vi "Color_Project.vi"() -> ()   [LabVIEW 2013]
uses:
  leitura de dados txt control.ctl
  <vilib>/Utility/file.llb/Write To Spreadsheet File (DBL).vi
panel:
  out "L*a*b* 3":dbl[](array[numeric])
  out "XYZ":dbl[](array[numeric])
  out "RGB":dbl[](array[numeric])
  in  "C0":dbl min=0.0 max=1.0
  in  "RMix1":dbl[](array[numeric])
  in  "Selected RGB":string="0"
  in  "RMix2":dbl[](array[numeric])
  in  "Reflectance":dbl[](array[numeric])
  in  "Tab Control":T1(tab)
  in  "Create reflectance":bool
  in  "Nome da cor":string
  in  "SaveReflectance":bool
  out "Reflectance graph":cluster{"Value":dbl[], dbl[]}(graph) caption="Espectro de reflectância selecionado"
  in  "CalculateColor":bool
  in  "SelectReflectance":bool
  out "CMF graph":cluster{"X":dbl[], "Y":dbl[]}[](graph)
  in  "Select Illuminant":T2
  in  "Color Matching Function":string(combo)
  out "Iluminante Graph":cluster{"Value":dbl[], "Value":dbl[]}[](graph)
  out "Color":u32(colorbox)
  in  "780nm":dbl(slide)=0.05 min=0.01 max=0.99 scale=0.0..1.0 scale format="%1.3f"
  in  "700nm":dbl(slide)=0.05 min=0.01 max=0.99 scale=0.0..1.0 scale format="%1.3f"
  in  "650nm":dbl(slide)=0.05 min=0.01 max=0.99 scale=0.0..1.0 scale format="%1.3f"
  in  "575nm":dbl(slide)=0.05 min=0.01 max=0.99 scale=0.0..1.0 scale format="%1.3f"
  in  "550nm":dbl(slide)=0.05 min=0.01 max=0.99 scale=0.0..1.0 scale format="%1.3f"
  in  "525nm":dbl(slide)=0.05 min=0.01 max=0.99 scale=0.0..1.0 scale format="%1.3f"
  in  "500nm":dbl(slide)=0.05 min=0.01 max=0.99 scale=0.0..1.0 scale format="%1.3f"
  in  "600nm":dbl(slide)=0.05 min=0.01 max=0.99 scale=0.0..1.0 scale format="%1.3f"
  in  "450nm":dbl(slide)=0.05 min=0.01 max=0.99 scale=0.0..1.0 scale format="%1.3f"
  in  "380nm":dbl(slide)=0.05 min=0.01 max=0.99 scale=0.0..1.0 scale format="%1.3f"
  in  "Tab Control 3":enum32{"Misturar", "Estatísticas"}(tab)
  out "ColorRM":cluster{"Value":dbl[], "Mixtured colors":dbl[]}(graph) caption="Gráfico da reflectância das cores misturadas"
  in  "MixColors":bool
  in  "Selecione a concentração da cor 1":dbl(slide) scale=0.0..1.0 scale format="%#.4g"
  out "2000":dbl caption="Diferença: Cor 1 - Cor misturada"
  out "CD2-M":dbl caption="Diferença: Cor 2 - Cor misturada"
  out "L*a*b* MixedColor":dbl[](array[numeric]) caption="L*a*b* mixtura"
  out "L*a*b*":dbl[](array[numeric]) caption="L*a*b* cor 1"
  out "L*a*b* 2":dbl[](array[numeric]) caption="L*a*b* cor 2"
  out "Cor complementar":u32(colorbox)
  out "MixedColors":u32(colorbox) caption="Cor resultante"
  out "ColorR2":cluster{"Value":dbl[], "Mixtured colors":dbl[]}(graph) caption="Gráfico de reflectância da cor 2"
  out "ColorR1":cluster{"Value":dbl[], "Mixtured colors":dbl[]}(graph) caption="Gráfico de reflectância da cor 1"
  out "Color2":u32(colorbox) caption="Cor selecionada"
  out "Color1":u32(colorbox) caption="Cor selecionada"
  in  "SelectColor2":bool
  in  "SelectColor1":bool
  in  "Color Matching Function 2":string(combo) caption="Selecione o CMF"
  in  "SelectIlluminant2":T2 caption="Selecione o iluminante"
  out "Color1Complementar":u32(colorbox) caption="Cor complementar"
  out "Cor complementar  2":u32(colorbox) caption="Cor complementar"
  in  "SelectColor2":bool
  in  "SelectColor1":bool
  in  "Tab Control 2":enum32{"L*", "a*", "b*"}(tab)
  out "Componente L*":cluster{"X":dbl[], "L*a*b intermediary":dbl[]}(graph)
  out "Componente a*":cluster{"X":dbl[], "L*a*b intermediary":dbl[]}(graph)
  out "Componente b*":cluster{"X":dbl[], "L*a*b intermediary":dbl[]}(graph)
  in  "Color Matching Function 3":string(combo) caption="Selecione o CMF"
  in  "SelectIlluminant2 2":T2 caption="Selecione o iluminante"
  in  "Colors":u32[](array[colorbox])
  out "Espectros de reflectância referentes as cores intermediárias obtidas":cluster{"X":dbl[], "Y":dbl[]}[](graph)
  in  "MixByConcentration":bool
  in  "Mixed":dbl[](array[numeric])
  in  "MixByColorDifference":bool
  out "Color1 2":u32
  out "Color2 2":u32
  in  "C1":dbl=0.1 min=0.0 max=1.0
  in  "DeltaLabel":string[](array[string]) caption="Delta E"
  in  "ConcentrationLabel":string[](array[string]) caption="Concentração"
  out "teste":i32[](array[numeric])
  out "IL Table":string[][](array[string])
  out "ILCols":i32
  out "ILRows":i32
  out "Selected illuminant value":dbl[](array[numeric])
  out "Is CMF selected?":bool
  out "Is illuminant selected?":bool
  out "CMF Table":string[][](array[string])
  out "NeedInterpolation?":bool
  out "WhiteReference":i32[](array[numeric])
  out "Intepoled iluminants":dbl[][](array[numeric])
  out "Selected\nCMF":dbl[][](array[numeric])
  out "cmf Index":dbl
  out "CMFCols":i32
  out "CMFRows":i32
  out "LambdaInterval":dbl[](array[numeric])
  out "Selected illuminant index":dbl
  out "Selected illuminant NV":cluster{"Value":string, dbl[]}
  # "Primeira etapa - Seleção da iluminação desejada"
  # "Segunda etapa - Seleção do estímulo ocular do observador"
  # "Terceira etapa - Seleção ou criação de espectros de reflectância"
  # "Selecione o CMF"
  # "Selecione o iluminante"
  # "Etapa final - Calcular cor referente aos espectros"
  # "Sistema para criação de espectros de reflectância"
  # "Etapa básica - Seleção de iluminação e estímulos oculares"
  # "Etapa final - Calcular a mistura das cores e dosar a concentração da cor referência"
  # "Segunda etapa - Selecionar as cores desejadas para efetuar a mistura"
  # "Desvios de cor"
  # "Coordenadas de cor"
  # "Nesta seção serão avaliadas diferentes maneiras para misturas de cores:\n1 - Por variação de concentração\n2 - Por variação de desvio de cor"
  # "Análise de variação das componentes L*a*b* das cores geradas"
  # "Seleção de componentes"
  # "Seleção do tipo da mistura a ser efetuado"
  # "Representação das cores intermediárias gerada a partir\ndas misturas,e seus respectivos desvios e concentrações"
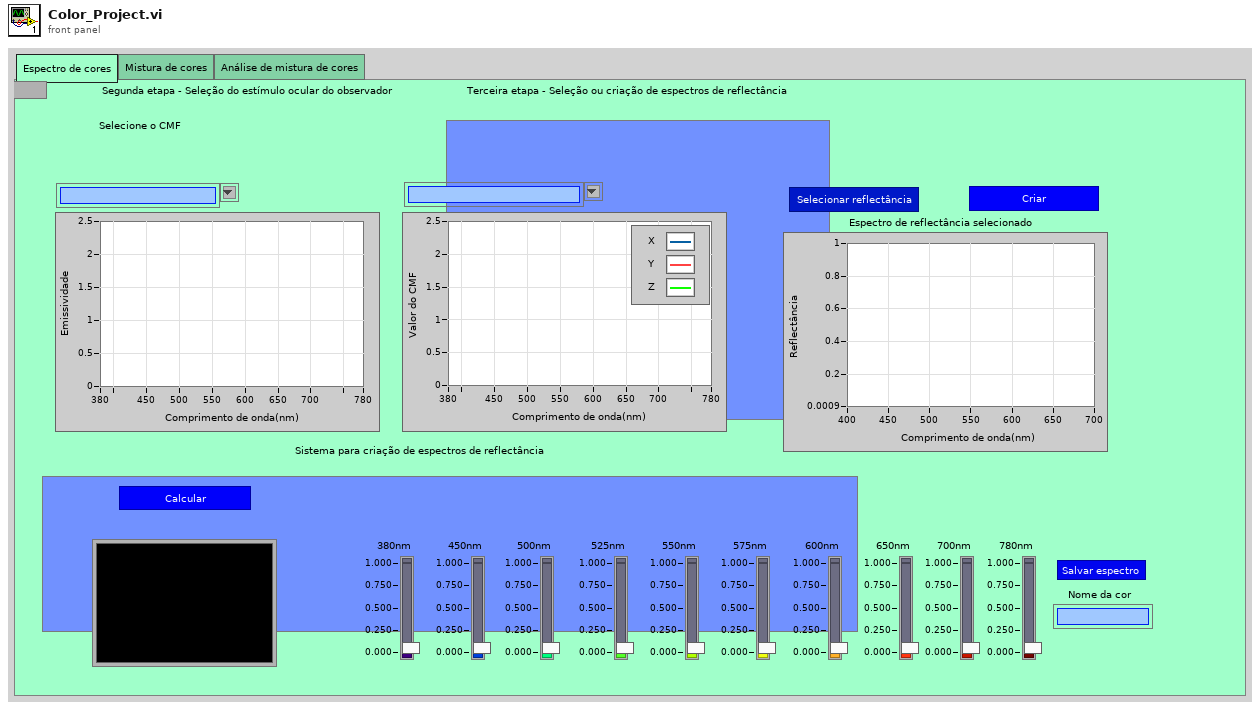
[diagram p1: front panel]
types:
  T1 = enum32{"Espectro de cores", "Mistura de cores", "Análise de mistura de cores"}
  T2 = typedef "leitura de dados txt control.ctl" = string
  T3 = cluster{"Value":cluster{"Value":string, dbl[]}, "Selected RGB":string, "Value":dbl[][]}
  T4 = cluster{"Color":u32, "RGB":dbl[], "L*a*b*":dbl[], "XYZ":dbl[]}
  T5 = cluster{cluster{i32[], dbl[]}, cluster{i32[], dbl[]}, cluster{i32[], dbl[]}}
  T6 = cluster{cluster{"X":dbl[], "L*a*b intermediary":dbl[]}, cluster{"X":dbl[], "L*a*b intermediary":dbl[]}, cluster{"X":dbl[], "L*a*b intermediary":dbl[]}}
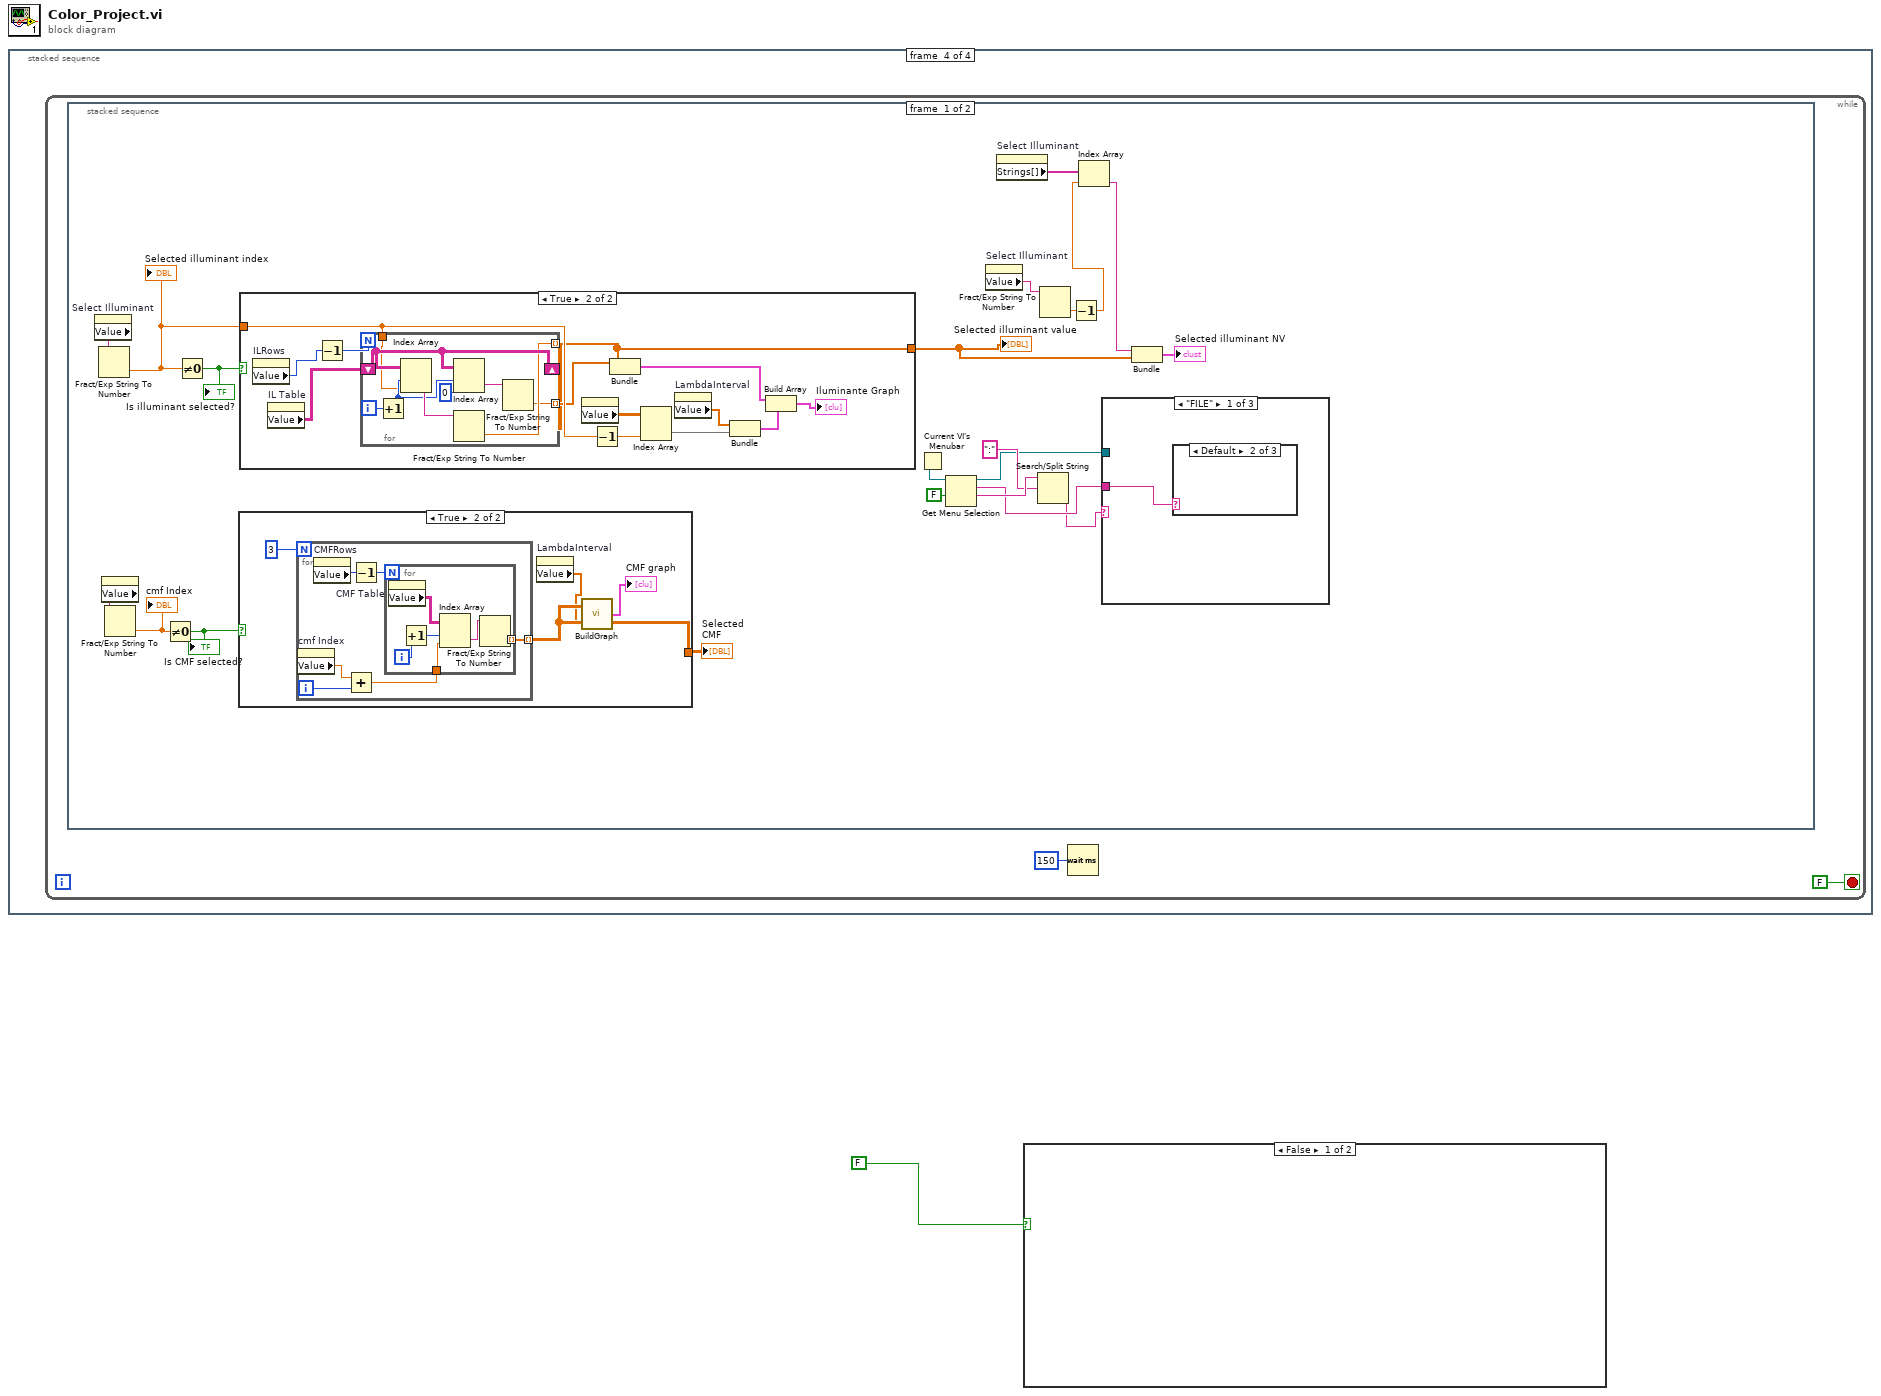
[diagram p0: block diagram]
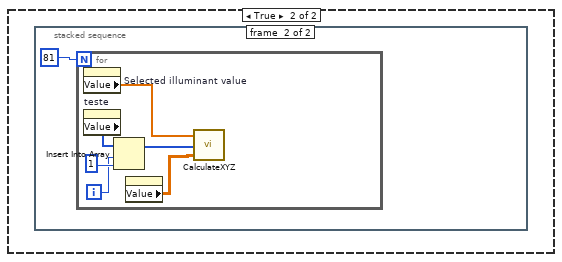
[diagram p2: hidden frame]
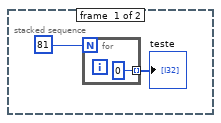
[diagram p3: hidden frame]
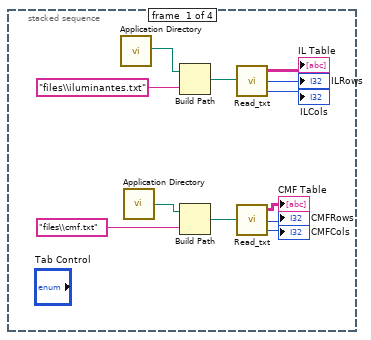
[diagram p4: hidden frame]
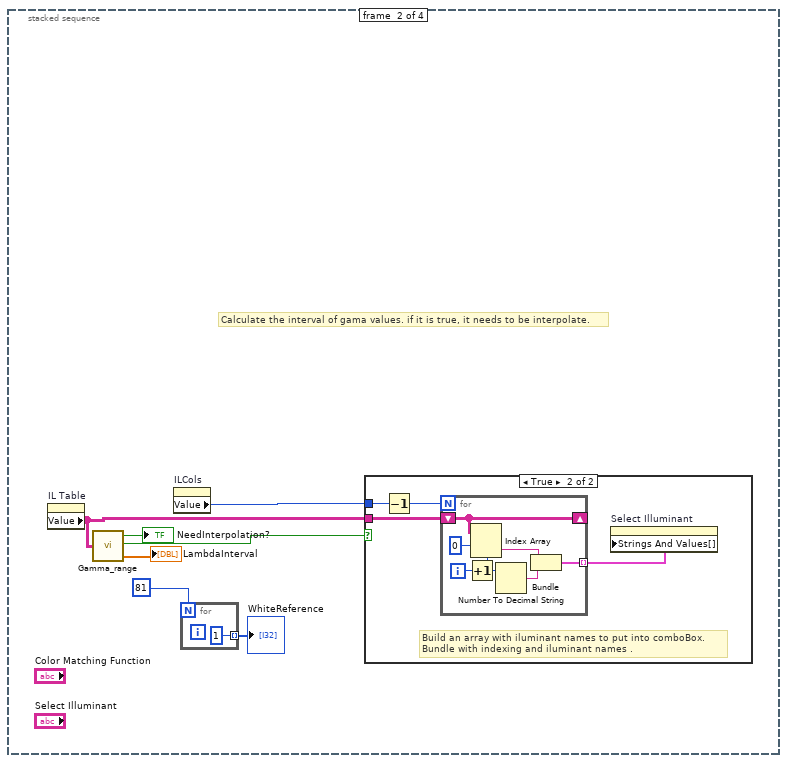
[diagram p5: hidden frame]
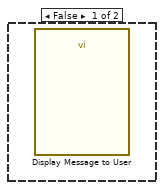
[diagram p6: hidden frame]
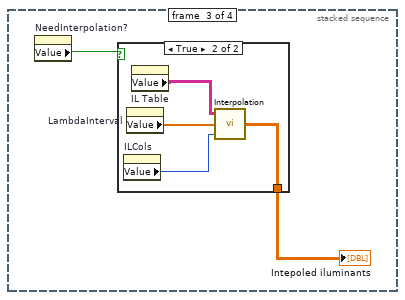
[diagram p7: hidden frame]
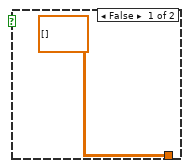
[diagram p8: hidden frame]
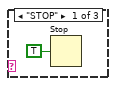
[diagram p9: hidden frame]
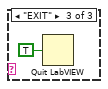
[diagram p10: hidden frame]
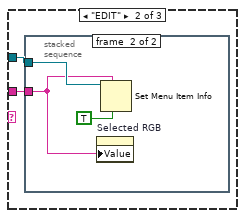
[diagram p11: hidden frame]
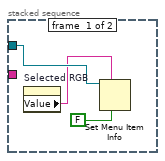
[diagram p12: hidden frame]
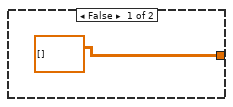
[diagram p14: hidden frame]
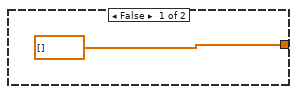
[diagram p15: hidden frame]
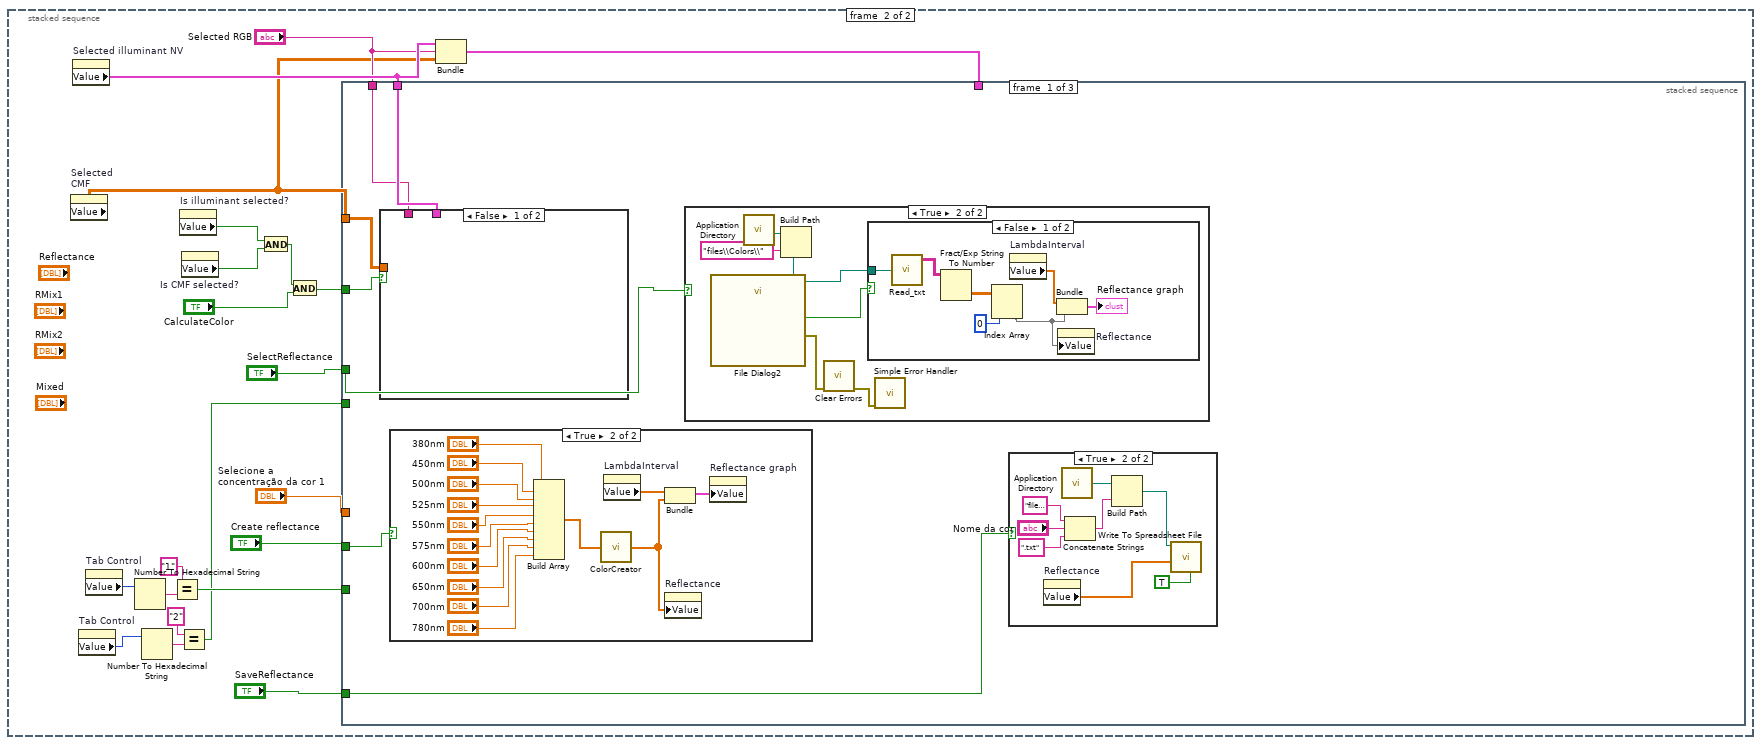
[diagram p16: hidden frame]
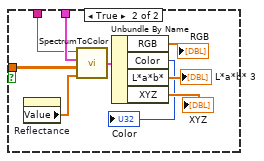
[diagram p18: hidden frame]
diagram:
  n1 = stacked-sequence {
    frame #0 {
      n2 = call <vilib>:"Application Directory.vi"() -> ("Application Directory"=w3:path)
      n3 = call <vilib>:"Application Directory.vi"() -> ("Application Directory"=w2:path)
      n4 = Build Path(base path=w3, name or relative path="files\\iluminantes.txt") -> (appended path=w5:path)
      n5 = Build Path(base path=w2, name or relative path="files\\cmf.txt") -> (appended path=w4:path)
      n6 = call "Read_txt.vi"("file path (dialog if empty)"=w5) -> ("Elements"=→"IL Table":string[][], "Rows"=→"ILRows":i32, "Cols"=→"ILCols":i32)
      n7 = call "Read_txt.vi"("file path (dialog if empty)"=w4) -> ("Elements"=→"CMF Table":string[][], "Rows"=→"CMFRows":i32, "Cols"=→"CMFCols":i32)
    }
    frame #1 {
      # "Calculate the interval of gama values. if it is true, it needs to be interpolate."
      n8 = property on="IL Table" class="Arr (strict)"() -> ("Value"=w15:string[][])  [unwired: 2 in, 2 out]
      n9 = call "Gamma_range.vi"("Illuminant Table"=w15) -> ("Interpolate"=→"NeedInterpolation?":bool, "In range?"=w17:bool, "GammaInterval"=→"LambdaInterval":dbl[])
      n10 = property on="ILCols" class="DigNum (strict)"() -> ("Value"=w18:i32)  [unwired: 2 in, 2 out]
      n11 = for {
        N: 81 -> [_]
        tunnel: [1] -> w19 mode=indexing
      }
      "WhiteReference" <- w19
      n12 = case shown="True" w17 {
        tunnel: w15 -> [_ w21]
        tunnel: w18 -> [_ w22]
        frame False {
          n13 = call "Display Message to User"() -> ()  [unwired: 10 in, 2 out]
        }
        frame True {
          # "Build an array with iluminant names to put into comboBox.\nBundle with indexing and iluminant names ."
          n14 = Decrement(x=w22) -> (x-1=w24:i32)
          n15 = for {
            N: w24 -> [_]
            shift-right: [w29] -> _
            shift-left: w21 -> [w29]
            tunnel: [w25] -> w23 mode=indexing
            i -> [w31]
            n16 = Increment(x=w31) -> (x+1=w28:i32)
            n17 = Index Array(array=w29, index (row)=0, index (col)=w28) -> (element=w26:string)
            n18 = Number To Decimal String(number=w28) -> (decimal integer string=w27:string)  [unwired: 1 in]
            n19 = Bundle("String"=w26, w27) -> (w25:cluster{"String":string, string})  [unwired: 1 in]
          }
          n20 = property on="Select Illuminant" class="CmbBox (strict)"("Strings And Values[]"=w23) -> ()  [unwired: 2 in, 2 out]
        }
      }
    }
    frame #2 {
      n21 = property on="NeedInterpolation?" class="Bool (strict)"() -> ("Value"=w34:bool)  [unwired: 2 in, 2 out]
      n22 = case shown="True" w34 {
        tunnel: [dbl[][] [] w38] -> w33
        frame False {
        }
        frame True {
          n23 = property on="ILCols" class="DigNum (strict)"() -> ("Value"=w36:i32)  [unwired: 2 in, 2 out]
          n24 = property on="LambdaInterval" class="Arr (strict)"() -> ("Value"=w39:dbl[])  [unwired: 2 in, 2 out]
          n25 = property on="IL Table" class="Arr (strict)"() -> ("Value"=w37:string[][])  [unwired: 2 in, 2 out]
          n26 = call "Interpolation.vi"("Number of Columns"=w36, "Lambda Interval"=w39, "Illuminants"=w37) -> ("Interpolated"=w38:dbl[][])
        }
      }
      "Intepoled iluminants" <- w33
    }
    frame #3 {
      n27 = while {
        stop <- FALSE stop-if-true
        n28 = stacked-sequence {
          frame #0 {
            n29 = property on="Select Illuminant" class="CmbBox (strict)"() -> ("Value"=w58:T2)  [unwired: 2 in, 2 out]
            n30 = Fract/Exp String To Number(string=w58) -> (number=w57:dbl)  [unwired: 3 in, 1 out]
            "Selected illuminant index" <- w57
            n31 = property on="Color Matching Function" class="CmbBox"() -> ("Value"=w60:string)  [unwired: 2 in, 2 out]
            n32 = Fract/Exp String To Number(string=w60) -> (number=w61:dbl)  [unwired: 3 in, 1 out]
            "cmf Index" <- w61
            n33 = Not Equal To 0?(x=w61) -> (x != 0?=w59:bool)
            "Is CMF selected?" <- w59
            n34 = Not Equal To 0?(x=w57) -> (x != 0?=w62:bool)
            "Is illuminant selected?" <- w62
            n35 = case shown="True" w59 {
              tunnel: [dbl[][] [] w77] -> w56
              frame False {
              }
              frame True {
                n36 = for {
                  N: 3 -> [_]
                  tunnel: [w81] -> w77 mode=indexing
                  i -> [w83]
                  n37 = property on="cmf Index" class="DigNum (strict)"() -> ("Value"=w84:dbl)  [unwired: 2 in, 2 out]
                  n38 = property on="CMFRows" class="DigNum (strict)"() -> ("Value"=w80:i32)  [unwired: 2 in, 2 out]
                  n39 = Add(x=w84, y=w83) -> (x+y=w82:dbl)
                  n40 = Decrement(x=w80) -> (x-1=w79:i32)
                  n41 = for {
                    N: w79 -> [_]
                    tunnel: w82 -> [w89]
                    tunnel: [w85] -> w81 mode=indexing
                    i -> [w88]
                    n42 = property on="CMF Table" class="Arr (strict)"() -> ("Value"=w90:string[][])  [unwired: 2 in, 2 out]
                    n43 = Increment(x=w88) -> (x+1=w87:i32)
                    n44 = Index Array(array=w90, index (row)=w87, index (col)=w89) -> (element=w86:string)
                    n45 = Fract/Exp String To Number(string=w86) -> (number=w85:dbl)  [unwired: 3 in, 1 out]
                  }
                }
                n46 = property on="LambdaInterval" class="Arr (strict)"() -> ("Value"=w76:dbl[])  [unwired: 2 in, 2 out]
                n47 = call "BuildGraph.vi"("X"=w76, "Y"=w77) -> ("Graph"=→"CMF graph":cluster{"X":dbl[], "Y":dbl[]}[])
              }
            }
            "Selected\nCMF" <- w56
            n48 = case shown="True" w62 {
              tunnel: w57 -> [_ w101]
              tunnel: [dbl[] [] w95] -> w55
              frame False {
              }
              frame True {
                n49 = property on="ILRows" class="DigNum (strict)"() -> ("Value"=w94:i32)  [unwired: 2 in, 2 out]
                n50 = property on="IL Table" class="Arr (strict)"() -> ("Value"=w93:string[][])  [unwired: 2 in, 2 out]
                n51 = Decrement(x=w94) -> (x-1=w104:i32)
                n52 = for {
                  N: w104 -> [_]
                  shift-right: [w112] -> _
                  shift-left: w93 -> [w112]
                  tunnel: w101 -> [w105]
                  tunnel: [w107] -> w95 mode=indexing
                  tunnel: [w106] -> w97 mode=indexing
                  i -> [w113]
                  n53 = Increment(x=w113) -> (x+1=w108:i32)
                  n54 = Index Array(array=w112, index (row)=w108, index (col)=w105) -> (element=w109:string)
                  n55 = Index Array(array=w112, index (row)=w108, index (col)=0 ("disabled index (col)")) -> (element=w110:string)
                  n56 = Fract/Exp String To Number(string=w109) -> (number=w107:dbl)  [unwired: 3 in, 1 out]
                  n57 = Fract/Exp String To Number(string=w110) -> (number=w106:dbl)  [unwired: 3 in, 1 out]
                }
                n58 = property on="Intepoled iluminants" class="Arr (strict)"() -> ("Value"=w99:dbl[][])  [unwired: 2 in, 2 out]
                n59 = Decrement(x=w101) -> (x-1=w100:dbl)
                n60 = Bundle(w97, w95) -> (w102:cluster{dbl[], dbl[]})  [unwired: 1 in]
                n61 = Index Array(array=w99, index (col)=w100) -> (element=w96:dbl[])  [unwired: 1 in]
                n62 = property on="LambdaInterval" class="Arr (strict)"() -> ("Value"=w98:dbl[])  [unwired: 2 in, 2 out]
                n63 = Bundle("Value"=w98, "Value"=w96) -> (w103:cluster{"Value":dbl[], "Value":dbl[]})  [unwired: 1 in]
                n64 = Build Array(w102, w103) -> (→"Iluminante Graph":cluster{"Value":dbl[], "Value":dbl[]}[])
              }
            }
            "Selected illuminant value" <- w55
            n65 = Current VI's Menubar() -> (w42:refnum<k9>)
            n66 = Get Menu Selection(0:w42, 2:FALSE ("block menu (F)")) -> (5:w45:refnum<k9>, 6:w44:string, 7:w47:string)  [unwired: 2 in, 2 out]
            n67 = property on="Select Illuminant" class="CmbBox (strict)"() -> ("Value"=w51:T2)  [unwired: 2 in, 2 out]
            n68 = property on="Select Illuminant" class="CmbBox (strict)"() -> ("Strings[]"=w53:string[])  [unwired: 2 in, 2 out]
            n69 = Search/Split String(string=w47, search string/char (-)=":") -> (substring before match=w43:string)  [unwired: 1 in, 2 out]
            n70 = Fract/Exp String To Number(string=w51) -> (number=w50:dbl)  [unwired: 3 in, 1 out]
            n71 = Decrement(x=w50) -> (x-1=w49:dbl)
            n72 = Index Array(array=w53, index=w49) -> (element=w52:string)
            n73 = case shown="\"FILE\"" w43 {
              tunnel: w45 -> [_ w67 _]
              tunnel: w44 -> [w63 w66 _]
              frame "FILE" {
                n74 = case shown="Default" w63 {
                  frame "STOP" {
                    n75 = Stop(stop? (T)=TRUE) -> ()
                  }
                  frame Default {
                  }
                  frame "EXIT" {
                    n76 = Quit LabVIEW(quit? (T)=TRUE) -> ()
                  }
                }
              }
              frame "EDIT" {
                n77 = stacked-sequence {
                  tunnel: w67 -> [w70 w73]
                  tunnel: w66 -> [_ w72]
                  frame #0 {
                    n78 = property on="Selected RGB" class="Str"() -> ("Value"=w68:string)  [unwired: 2 in, 2 out]
                    n79 = Set Menu Item Info(6:FALSE ("enabled"), 7:w68, 11:w70) -> ()  [unwired: 4 in, 2 out]
                  }
                  frame #1 {
                    n80 = property on="Selected RGB" class="Str"("Value"=w72) -> ()  [unwired: 2 in, 2 out]
                    n81 = Set Menu Item Info(6:TRUE ("enabled"), 7:w72, 11:w73) -> ()  [unwired: 4 in, 2 out]
                  }
                }
              }
              frame Default {
              }
            }
            n82 = Bundle(w52, w55) -> (→"Selected illuminant NV":cluster{string, dbl[]})  [unwired: 1 in]
          }
          frame #1 {
            n83 = property on="Selected\nCMF" class="Arr (strict)"() -> ("Value"=w125:dbl[][])  [unwired: 2 in, 2 out]
            n84 = property on="Selected illuminant NV" class="Clust (strict)"() -> ("Value"=w127:cluster{"Value":string, dbl[]})  [unwired: 2 in, 2 out]
            n85 = property on="Tab Control" class="TabCtl (strict)"() -> ("Value"=w118:T1)  [unwired: 2 in, 2 out]
            n86 = property on="Tab Control" class="TabCtl (strict)"() -> ("Value"=w121:T1)  [unwired: 2 in, 2 out]
            n87 = Number To Hexadecimal String(2:w121) -> (0:w122:string)  [unwired: 1 in]
            n88 = Number To Hexadecimal String(2:w118) -> (0:w119:string)  [unwired: 1 in]
            n89 = Equal?(x="1", y=w122) -> (x = y?=w120:bool)
            n90 = Equal?(x="2", y=w119) -> (x = y?=w116:bool)
            n91 = property on="Is illuminant selected?" class="Bool (strict)"() -> ("Value"=w132:bool)  [unwired: 2 in, 2 out]
            n92 = property on="Is CMF selected?" class="Bool (strict)"() -> ("Value"=w133:bool)  [unwired: 2 in, 2 out]
            n93 = And(x=w132, y=w133) -> (x .and. y?=w114:bool)
            n94 = And(x=w114, y="CalculateColor") -> (x .and. y?=w131:bool)
            n95 = Bundle("Value"=w127, "Selected RGB"="Selected RGB", "Value"=w125) -> (w124:T3)  [unwired: 1 in]
            n96 = stacked-sequence {
              tunnel: w127 -> [w139 w189 w248]
              tunnel: w125 -> [w138 w188 w247]
              tunnel: w131 -> [w137 _ _]
              tunnel: "SelectReflectance" -> [w141 _ _]
              tunnel: "Create reflectance" -> [w140 _ _]
              tunnel: "Selected RGB" -> [w136 w190 w249]
              tunnel: "Selecione a concentração da cor 1" -> [_ w191 _]
              tunnel: "SaveReflectance" -> [w135 _ _]
              tunnel: w124 -> [_ _ w246]
              tunnel: w120 -> [_ w187 _]
              tunnel: w116 -> [_ _ w245]
              frame #0 {
                n97 = case shown="False" w137 {
                  tunnel: w139 -> [_ w157]
                  tunnel: w138 -> [_ w156]
                  tunnel: w136 -> [_ w154]
                  frame False {
                  }
                  frame True {
                    n98 = property on="Reflectance" class="Arr (strict)"() -> ("Value"=w155:dbl[])  [unwired: 2 in, 2 out]
                    n99 = call "SpectrumToColor.vi"("Reflectance"=w155, "CMF"=w156, "Illuminant"=w157, "Selected RGB"=w154) -> ("Color,XYZ,RGB,Lab"=w158:T4)
                    n100 = Unbundle By Name(w158) -> ("RGB"=→"RGB":dbl[], "Color"=→"Color":u32, "L*a*b*"=→"L*a*b* 3":dbl[], "XYZ"=→"XYZ":dbl[])
                  }
                }
                n101 = case shown="True" w140 {
                  frame False {
                  }
                  frame True {
                    n102 = Build Array("380nm", "450nm", "500nm", "525nm", "550nm", "575nm", "600nm", "650nm", "700nm", "780nm") -> (w162:dbl[])
                    n103 = call "ColorCreator.vi"("Reflectance values"=w162) -> ("Spectrum"=w159:dbl[])
                    n104 = property on="LambdaInterval" class="Arr (strict)"() -> ("Value"=w160:dbl[])  [unwired: 2 in, 2 out]
                    n105 = Bundle("Value"=w160, "Spectrum"=w159) -> (w161:cluster{"Value":dbl[], "Spectrum":dbl[]})  [unwired: 1 in]
                    n106 = property on="Reflectance" class="Arr (strict)"("Value"=w159) -> ()  [unwired: 2 in, 2 out]
                    n107 = property on="Reflectance graph" class="XYGraph (strict)"("Value"=w161) -> ()  [unwired: 2 in, 2 out]
                  }
                }
                n108 = case shown="True" w141 {
                  frame False {
                  }
                  frame True {
                    n109 = call <vilib>:"Application Directory.vi"() -> ("Application Directory"=w178:path)
                    n110 = Build Path(base path=w178, name or relative path="files\\Colors\\") -> (appended path=w177:path)
                    n111 = call "File Dialog2"("start path"=w177) -> ("selected path"=w175:path, "cancelled"=w176:bool, "error out"=w174:errorcluster)  [unwired: 11 in, 1 out]
                    n112 = call <vilib>:"Clear Errors.vi"("error in (no error)"=w174) -> ("error out"=w173:errorcluster)  [unwired: 6 in]
                    n113 = case shown="False" w176 {
                      tunnel: w175 -> [w181 _]
                      frame False {
                        n114 = call "Read_txt.vi"("file path (dialog if empty)"=w181) -> ("Elements"=w186:string[][])  [unwired: 2 out]
                        n115 = Fract/Exp String To Number(string=w186) -> (number=w185:dbl[][])  [unwired: 3 in, 1 out]
                        n116 = Index Array(array=w185, index (col)=0 ("index (row)")) -> (element=w180:dbl[])  [unwired: 1 in]
                        n117 = property on="LambdaInterval" class="Arr (strict)"() -> ("Value"=w183:dbl[])  [unwired: 2 in, 2 out]
                        n118 = Bundle("Value"=w183, w180) -> (→"Reflectance graph":cluster{"Value":dbl[], dbl[]})  [unwired: 1 in]
                        n119 = property on="Reflectance" class="Arr (strict)"("Value"=w180) -> ()  [unwired: 2 in, 2 out]
                      }
                      frame True {
                        n120 = call "Display Message to User2"() -> ()  [unwired: 10 in, 2 out]
                      }
                    }
                    n121 = call <vilib>:"Simple Error Handler.vi"("error in (no error)"=w173) -> ()  [unwired: 4 in, 5 out]
                  }
                }
                n122 = case shown="True" w135 {
                  frame False {
                  }
                  frame True {
                    n123 = property on="Reflectance" class="Arr (strict)"() -> ("Value"=w147:dbl[])  [unwired: 2 in, 2 out]
                    n124 = call <vilib>:"Application Directory.vi"() -> ("Application Directory"=w149:path)
                    n125 = Concatenate Strings("files\\Colors\\" ("name or relative path"), "Nome da cor", ".txt") -> (w143:string)
                    n126 = Build Path(base path=w149, name or relative path=w143) -> (appended path=w148:path)
                    n127 = call-poly <vilib>:"Write To Spreadsheet File.vi"("transpose? (no:F)"=TRUE, "1D data"=w147, "file path (dialog if empty)"=w148) -> ()  [unwired: 5 in, 1 out]
                  }
                }
              }
              frame #1 {
                n128 = case shown="True" w187 {
                  tunnel: w191 -> [_ w206]
                  tunnel: w190 -> [_ w205]
                  tunnel: w189 -> [_ w204]
                  tunnel: w188 -> [_ w203]
                  frame False {
                  }
                  frame True {
                    n129 = property on="Color Matching Function" class="CmbBox"("Value"="Color Matching Function 2") -> ()  [unwired: 2 in, 2 out]
                    n130 = case shown="True" "MixColors" {
                      tunnel: w206 -> [_ w221]
                      frame False {
                      }
                      frame True {
                        n131 = property on="RMix2" class="Arr (strict)"() -> ("Value"=w222:dbl[])  [unwired: 2 in, 2 out]
                        n132 = property on="RMix1" class="Arr (strict)"() -> ("Value"=w211:dbl[])  [unwired: 2 in, 2 out]
                        n133 = call "ColorMixture.vi"("Concentration1"=w221, "Reflectance spectrum 2"=w222, "Reflectance spectrum"=w211) -> ("Mixtured colors"=w216:dbl[])  [unwired: 1 in]
                        n134 = property on="Selected illuminant NV" class="Clust (strict)"() -> (error out=w214:errorcluster, "Value"=w220:cluster{"Value":string, dbl[]})  [unwired: 2 in, 1 out]
                        n135 = property on="Selected\nCMF" class="Arr (strict)"() -> ("Value"=w219:dbl[][])  [unwired: 2 in, 2 out]
                        n136 = property on="LambdaInterval" class="Arr (strict)"() -> ("Value"=w217:dbl[])  [unwired: 2 in, 2 out]
                        n137 = property on="Selected RGB" class="Str"(error in=w214) -> ("Value"=w213:string)  [unwired: 1 in, 2 out]
                        n138 = call "SpectrumToColor.vi"("Reflectance"=w216, "CMF"=w219, "Illuminant"=w220, "Selected RGB"=w213) -> ("Color,XYZ,RGB,Lab"=w218:T4)
                        n139 = Bundle("Value"=w217, "Mixtured colors"=w216) -> (→"ColorRM":cluster{"Value":dbl[], "Mixtured colors":dbl[]})  [unwired: 1 in]
                        n140 = Unbundle By Name(w218) -> ("Color"=w208:u32, "L*a*b*"=→"L*a*b* MixedColor":dbl[], "RGB"=w210:dbl[])
                        "MixedColors" <- w208
                        n141 = call "RGBtoComplementar.vi"("RGB"=w210) -> ("Complementar"=→"Cor complementar":u32)
                        n142 = property on="Selecione a concentração da cor 1" class="Slide (strict)"("Fill Color"=w208) -> ()  [unwired: 2 in, 2 out]
                      }
                    }
                    n143 = case shown="True" "SelectColor1" {
                      tunnel: w205 -> [_ w243]
                      tunnel: w204 -> [_ w242]
                      tunnel: w203 -> [_ w241]
                      frame False {
                      }
                      frame True {
                        n144 = call "SelectColor.vi"("CMF"=w241, "Illuminant"=w242, "Selected RGB"=w243) -> ("Reflectance"=w236:dbl[], "Color,XYZ,RGB,Lab"=w240:T4)
                        n145 = property on="RMix1" class="Arr (strict)"("Value"=w236) -> ()  [unwired: 2 in, 2 out]
                        n146 = property on="LambdaInterval" class="Arr (strict)"() -> ("Value"=w238:dbl[])  [unwired: 2 in, 2 out]
                        n147 = Unbundle By Name(w240) -> ("L*a*b*"=→"L*a*b*":dbl[], "Color"=→"Color1":u32, "RGB"=w235:dbl[])
                        n148 = Bundle("Value"=w238, "Reflectance"=w236) -> (→"ColorR1":cluster{"Value":dbl[], "Reflectance":dbl[]})  [unwired: 1 in]
                        n149 = call "RGBtoComplementar.vi"("RGB"=w235) -> ("Complementar"=→"Color1Complementar":u32)
                      }
                    }
                    n150 = case shown="True" "SelectColor2" {
                      tunnel: w205 -> [_ w233]
                      tunnel: w204 -> [_ w232]
                      tunnel: w203 -> [_ w231]
                      frame False {
                      }
                      frame True {
                        n151 = call "SelectColor.vi"("CMF"=w231, "Illuminant"=w232, "Selected RGB"=w233) -> ("Reflectance"=w226:dbl[], "Color,XYZ,RGB,Lab"=w229:T4)
                        n152 = Unbundle By Name(w229) -> ("L*a*b*"=→"L*a*b* 2":dbl[], "Color"=→"Color2":u32, "RGB"=w224:dbl[])
                        n153 = property on="RMix2" class="Arr (strict)"("Value"=w226) -> ()  [unwired: 2 in, 2 out]
                        n154 = property on="LambdaInterval" class="Arr (strict)"() -> ("Value"=w227:dbl[])  [unwired: 2 in, 2 out]
                        n155 = Bundle("Value"=w227, "Reflectance"=w226) -> (→"ColorR2":cluster{"Value":dbl[], "Reflectance":dbl[]})  [unwired: 1 in]
                        n156 = call "RGBtoComplementar.vi"("RGB"=w224) -> ("Complementar"=→"Cor complementar  2":u32)
                      }
                    }
                    n157 = property on="Select Illuminant" class="CmbBox (strict)"("Value"="SelectIlluminant2") -> ()  [unwired: 2 in, 2 out]
                    n158 = property on="L*a*b* MixedColor" class="Arr (strict)"() -> ("Value"=w197:dbl[])  [unwired: 2 in, 2 out]
                    n159 = property on="L*a*b*" class="Arr (strict)"() -> ("Value"=w199:dbl[])  [unwired: 2 in, 2 out]
                    n160 = property on="L*a*b* 2" class="Arr (strict)"() -> ("Value"=w198:dbl[])  [unwired: 2 in, 2 out]
                    n161 = Bundle("Value"=w198, "Value"=w197) -> (w194:cluster{"Value":dbl[], "Value":dbl[]})  [unwired: 1 in]
                    n162 = Bundle("Value"=w199, "Value"=w197) -> (w193:cluster{"Value":dbl[], "Value":dbl[]})  [unwired: 1 in]
                    n163 = call "DeltaE(2000).vi"("L*a*b Colors"=w194) -> ("Delta E"=→"CD2-M":dbl)
                    n164 = call "DeltaE(2000).vi"("L*a*b Colors"=w193) -> ("Delta E"=→"2000":dbl)
                  }
                }
              }
              frame #2 {
                n165 = case shown="True" w245 {
                  tunnel: w249 -> [_ w261]
                  tunnel: w248 -> [_ w260]
                  tunnel: w247 -> [_ w259]
                  tunnel: w246 -> [_ w258]
                  frame False {
                  }
                  frame True {
                    n166 = case shown="True" "MixByConcentration" {
                      tunnel: w261 -> [_ w387]
                      tunnel: w260 -> [_ w386]
                      tunnel: w259 -> [_ w385]
                      frame False {
                      }
                      frame True {
                        n167 = property on="LambdaInterval" class="Arr (strict)"() -> ("Value"=w383:dbl[])  [unwired: 2 in, 2 out]
                        n168 = for {
                          N: 11 -> [_]
                          tunnel: w387 -> [w397]
                          tunnel: w386 -> [w396]
                          tunnel: w385 -> [w395]
                          tunnel: [w393] -> w379 mode=indexing
                          tunnel: [w392] -> w384 mode=indexing
                          tunnel: [w391] -> w380 mode=indexing
                          tunnel: [w389] -> w373 mode=indexing
                          i -> [w390]
                          n169 = property on="RMix1" class="Arr (strict)"() -> ("Value"=w399:dbl[])  [unwired: 2 in, 2 out]
                          n170 = property on="RMix2" class="Arr (strict)"() -> ("Value"=w398:dbl[])  [unwired: 2 in, 2 out]
                          n171 = Divide(x=w390, y=10) -> (x/y=w391:dbl)
                          n172 = call "ColorMixture.vi"("Concentration1"=w391, "Reflectance spectrum 2"=w398, "Reflectance spectrum"=w399) -> ("Mixtured colors"=w392:dbl[])  [unwired: 1 in]
                          n173 = call "SpectrumToColor.vi"("Reflectance"=w392, "CMF"=w395, "Illuminant"=w396, "Selected RGB"=w397) -> ("Color,XYZ,RGB,Lab"=w394:T4)
                          n174 = Unbundle By Name(w394) -> ("Color"=w393:u32, "L*a*b*"=w389:dbl[])
                        }
                        n175 = call "BuildGraph.vi"("X"=w383, "Y"=w384) -> ("Graph"=w382:cluster{"X":dbl[], "Y":dbl[]}[])
                        n176 = property on="Espectros de reflectância referentes as cores intermediárias obtidas" class="XYGraph (strict)"("Value"=w382) -> ()  [unwired: 2 in, 2 out]
                        n177 = Number To Fractional String(number=w380, precision (6)=i16 2) -> (F-format string=w374:string[])  [unwired: 2 in]
                        n178 = property on="Colors" class="Arr (strict)"("Value"=w379) -> ()  [unwired: 2 in, 2 out]
                        n179 = call "LabConcentrationGraph.vi"("L*a*b*"=w373) -> ("L*a*b Variation"=w378:T5)
                        n180 = call "BuildDeltaString.vi"("L*a*b"=w373) -> ("DeltaEString"=w372:string[])
                        n181 = property on="ConcentrationLabel" class="Arr (strict)"("Value"=w374) -> ()  [unwired: 2 in, 2 out]
                        n182 = Unbundle(w378) -> (w377:cluster{i32[], dbl[]}, w376:cluster{i32[], dbl[]}, w375:cluster{i32[], dbl[]})
                        n183 = property on="DeltaLabel" class="Arr (strict)"("Value"=w372) -> ()  [unwired: 2 in, 2 out]
                        n184 = property on="Componente L*" class="XYGraph (strict)"("Value"=w377) -> ()  [unwired: 2 in, 2 out]
                        n185 = property on="Componente b*" class="XYGraph (strict)"("Value"=w376) -> ()  [unwired: 2 in, 2 out]
                        n186 = property on="Componente a*" class="XYGraph (strict)"("Value"=w375) -> ()  [unwired: 2 in, 2 out]
                      }
                    }
                    n187 = property on="RMix2" class="Arr (strict)"() -> (error out=w256:errorcluster, "Value"=w257:dbl[])  [unwired: 2 in, 1 out]
                    n188 = property on="Select Illuminant" class="CmbBox (strict)"("Value"="SelectIlluminant2 2") -> ()  [unwired: 2 in, 2 out]
                    n189 = property on="Color Matching Function" class="CmbBox"("Value"="Color Matching Function 3") -> ()  [unwired: 2 in, 2 out]
                    n190 = property on="Mixed" class="Arr (strict)"(error in=w256, "Value"=w257) -> ()  [unwired: 1 in, 2 out]
                    n191 = case shown="True" "SelectColor2" {
                      frame False {
                      }
                      frame True {
                        n192 = call "FileToDoubleArray.vi"() -> ("Reflectance"=w262:dbl[])
                        n193 = property on="RMix2" class="Arr (strict)"("Value"=w262) -> ()  [unwired: 2 in, 2 out]
                      }
                    }
                    n194 = case shown="True" "SelectColor1" {
                      frame False {
                      }
                      frame True {
                        n195 = call "FileToDoubleArray.vi"() -> ("Reflectance"=w263:dbl[])
                        n196 = property on="RMix1" class="Arr (strict)"("Value"=w263) -> ()  [unwired: 2 in, 2 out]
                      }
                    }
                    n197 = case shown="True" "MixByColorDifference" {
                      tunnel: w258 -> [_ w276]
                      frame False {
                      }
                      frame True {
                        n198 = property on="C0" class="DigNum (strict)"("Value"=0.0 ("C0")) -> ()  [unwired: 2 in, 2 out]
                        n199 = property on="C1" class="DigNum (strict)"("Value"=0.1 ("C1")) -> ()  [unwired: 2 in, 2 out]
                        n200 = flat-sequence {
                          tunnel: w276 -> [w289]
                          tunnel: [w287] -> w273
                          tunnel: [w286] -> w272
                          tunnel: [w285] -> w271
                          tunnel: [w284] -> w270
                          tunnel: [w283] -> w269
                          tunnel: [w282] -> w268
                          tunnel: [w281] -> w267
                          tunnel: [w280] -> w266
                          tunnel: [w279] -> w265
                          tunnel: [w277] -> w264
                          tunnel: w273 -> [w363]
                          tunnel: w272 -> [w364]
                          tunnel: w271 -> [w360]
                          tunnel: w270 -> [w359]
                          tunnel: w269 -> [w354]
                          tunnel: w268 -> [w353]
                          tunnel: w267 -> [w351]
                          tunnel: w266 -> [w347]
                          tunnel: w265 -> [w336]
                          tunnel: w264 -> [w331]
                          frame #0 {
                            # "dE"
                            n201 = property on="RMix1" class="Arr (strict)"() -> ("Value"=w283:dbl[])  [unwired: 2 in, 2 out]
                            n202 = property on="RMix2" class="Arr (strict)"() -> ("Value"=w282:dbl[])  [unwired: 2 in, 2 out]
                            n203 = call "SpectrumDeltaE.vi"("Iluminant - RGB - CMF"=w289, "Reflectance 2"=w282, "Reflectance 1"=w283) -> ("Color1"=w287:T4, "Delta E"=w290:dbl, "Color2"=w286:T4)  [unwired: 1 in]
                            n204 = Divide(x=w290, y=10.0) -> (x/y=w288:dbl)
                            n205 = for {
                              N: 9 -> [_]
                              tunnel: w283 -> [w301]
                              tunnel: w282 -> [w300]
                              tunnel: w289 -> [w299]
                              tunnel: w288 -> [w298]
                              tunnel: [w296] -> w284 mode=indexing
                              tunnel: [w295] -> w285 mode=indexing
                              tunnel: [w294] -> w281 mode=indexing
                              tunnel: [w293] -> w280
                              tunnel: [w293] -> w279 mode=indexing
                              tunnel: [w292] -> w277 mode=indexing
                              n206 = while {
                                tunnel: w301 -> [w322]
                                tunnel: w300 -> [w321]
                                tunnel: w299 -> [w319]
                                tunnel: w298 -> [w314]
                                tunnel: [w308] -> w297
                                tunnel: [w305] -> w296
                                tunnel: [w303] -> w294
                                tunnel: [w302] -> w292
                                i -> [w306]
                                stop <- w309 stop-if-true
                                n207 = property on="C1" class="DigNum (strict)"() -> ("Value"=w302:dbl)  [unwired: 2 in, 2 out]
                                n208 = property on="Mixed" class="Arr (strict)"() -> ("Value"=w320:dbl[])  [unwired: 2 in, 2 out]
                                n209 = Multiply(x=w314, y=1.01) -> (x*y=w316:dbl)
                                n210 = Multiply(x=w314, y=0.91) -> (x*y=w313:dbl)
                                n211 = Less?(x=10, y=w306) -> (x < y?=w318:bool)
                                n212 = call "ColorMixture.vi"("Concentration1"=w302, "Reflectance spectrum 2"=w321, "Reflectance spectrum"=w322) -> ("Mixtured colors"=w305:dbl[])  [unwired: 1 in]
                                n213 = call "SpectrumDeltaE.vi"("Iluminant - RGB - CMF"=w319, "Reflectance 2"=w320, "Reflectance 1"=w305) -> ("Color1"=w308:T4, "Delta E"=w303:dbl)  [unwired: 1 in, 1 out]
                                n214 = Greater?(x=w303, y=w316) -> (0:w307:bool)
                                n215 = Less?(x=w303, y=w313) -> (x < y?=w312:bool)
                                n216 = Or(x=w307, y=w312) -> (x .or. y?=w310:bool)
                                n217 = case shown="True" w310 {
                                tunnel: w303 -> [_ _]
                                tunnel: w307 -> [_ w323]
                                frame False {
                                }
                                frame True {
                                n218 = case shown="False" w323 {
                                frame False {
                                n219 = stacked-sequence {
                                frame #0 {
                                n220 = property on="C1" class="DigNum (strict)"() -> ("Value"=w324:dbl)  [unwired: 2 in, 2 out]
                                n221 = property on="C0" class="DigNum (strict)"("Value"=w324) -> ()  [unwired: 2 in, 2 out]
                                }
                                frame #1 {
                                n222 = property on="C1" class="DigNum (strict)"() -> ("Value"=w326:dbl)  [unwired: 2 in, 2 out]
                                n223 = formula code="C1=C1*1.5;\nif(C1 > 1)\nC1 = 0.99;"("C1"=w326) -> ("C1"=w325:dbl)
                                n224 = property on="C1" class="DigNum (strict)"("Value"=w325) -> ()  [unwired: 2 in, 2 out]
                                }
                                }
                                }
                                frame True {
                                n225 = property on="C0" class="DigNum (strict)"() -> ("Value"=w328:dbl)  [unwired: 2 in, 2 out]
                                n226 = property on="C1" class="DigNum (strict)"() -> ("Value"=w329:dbl)  [unwired: 2 in, 2 out]
                                n227 = formula code="C1 = (C1+C0)/2;\nif(C1 > 1)\nC1 = 0.99;"("C1"=w329, "C0"=w328) -> ("C1"=w327:dbl)
                                n228 = property on="C1" class="DigNum (strict)"("Value"=w327) -> ()  [unwired: 2 in, 2 out]
                                }
                                }
                                }
                                }
                                n229 = Not(x=w310) -> (.not. x?=w311:bool)
                                n230 = Or(x=w311, y=w318) -> (x .or. y?=w309:bool)
                              }
                              n231 = property on="Mixed" class="Arr (strict)"("Value"=w296) -> ()  [unwired: 2 in, 2 out]
                              n232 = Unbundle(w297) -> ("Color"=w295:u32, "L*a*b*"=w293:dbl[])  [unwired: 2 out]
                            }
                          }
                          frame #1 {
                            n233 = property on="Color1" class="DigNum (strict)"() -> ("Value"=w370:u32)  [unwired: 2 in, 2 out]
                            n234 = property on="Color2" class="DigNum (strict)"() -> ("Value"=w371:u32)  [unwired: 2 in, 2 out]
                            n235 = Unbundle By Name(w364) -> ("Color"=→"Color2 2":u32, "L*a*b*"=w337:dbl[])
                            n236 = Unbundle By Name(w363) -> ("Color"=→"Color1 2":u32, "L*a*b*"=w338:dbl[])
                            n237 = Insert Into Array(array=w359, index (row)=0, new element=w354) -> (w355:dbl[][])  [unwired: 1 in]
                            n238 = Insert Into Array(array=w355, index (row)=10, new element=w353) -> (w357:dbl[][])  [unwired: 1 in]
                            n239 = Number To Fractional String(number=w351, precision (6)=i16 2) -> (F-format string=w350:string[])  [unwired: 2 in]
                            n240 = call "BuildConcentrationString.vi"("Concentrations"=w331) -> ("Concentration String"=w330:string[])
                            n241 = Insert Into Array(array=w360, index=0, new element=w370) -> (w368:u32[])
                            n242 = Insert Into Array(array=w368, index=10, new element=w371) -> (w361:u32[])
                            n243 = property on="LambdaInterval" class="Arr (strict)"() -> ("Value"=w339:dbl[])  [unwired: 2 in, 2 out]
                            n244 = property on="Colors" class="Arr (strict)"("Value"=w361) -> ()  [unwired: 2 in, 2 out]
                            n245 = property on="ConcentrationLabel" class="Arr (strict)"("Value"=w330) -> ()  [unwired: 2 in, 2 out]
                            n246 = Insert Into Array(array=w350, index=0, new element="0" ("new element/subarray")) -> (w342:string[])
                            n247 = call "BuildGraph.vi"("X"=w339, "Y"=w357) -> ("Graph"=w362:cluster{"X":dbl[], "Y":dbl[]}[])
                            n248 = call "BuildLabDeltaGraph.vi"("L*a*b intermediary"=w336, "L*a*b 2"=w337, "L*a*b 1"=w338) -> ("L*a*b* Graphs"=w335:T6)
                            n249 = Bundle("L*a*b*"=w338, "L*a*b*"=w347) -> (w346:cluster{"L*a*b*":dbl[], "L*a*b*":dbl[]})  [unwired: 1 in]
                            n250 = property on="Espectros de reflectância referentes as cores intermediárias obtidas" class="XYGraph (strict)"("Value"=w362) -> ()  [unwired: 2 in, 2 out]
                            n251 = call "DeltaE(2000).vi"("L*a*b Colors"=w346) -> ("Delta E"=w344:dbl)
                            n252 = Number To Fractional String(number=w344, precision (6)=i16 2) -> (F-format string=w340:string)  [unwired: 2 in]
                            n253 = Insert Into Array(array=w342, index=10, new element=w340) -> (w341:string[])
                            n254 = property on="DeltaLabel" class="Arr (strict)"("Value"=w341) -> ()  [unwired: 2 in, 2 out]
                            n255 = Unbundle(w335) -> (w334:cluster{"X":dbl[], "L*a*b intermediary":dbl[]}, w333:cluster{"X":dbl[], "L*a*b intermediary":dbl[]}, w332:cluster{"X":dbl[], "L*a*b intermediary":dbl[]})
                            n256 = property on="Componente L*" class="XYGraph (strict)"("Value"=w334) -> ()  [unwired: 2 in, 2 out]
                            n257 = property on="Componente b*" class="XYGraph (strict)"("Value"=w333) -> ()  [unwired: 2 in, 2 out]
                            n258 = property on="Componente a*" class="XYGraph (strict)"("Value"=w332) -> ()  [unwired: 2 in, 2 out]
                          }
                        }
                      }
                    }
                  }
                }
              }
            }
          }
        }
        n259 = Wait (ms)(milliseconds to wait=u32 150) -> ()  [unwired: 1 out]
      }
    }
  }
  n260 = case shown="False" FALSE {
    frame False {
    }
    frame True {
      n261 = stacked-sequence {
        frame #0 {
          n262 = for {
            N: 81 -> [_]
            tunnel: [0] -> w401 mode=indexing
          }
          "teste" <- w401
        }
        frame #1 {
          n263 = for {
            N: 81 -> [_]
            i -> [w409]
            n264 = property on="Selected illuminant value" class="Arr (strict)"() -> ("Value"=w407:dbl[])  [unwired: 2 in, 2 out]
            n265 = property on="teste" class="Arr (strict)"() -> ("Value"=w408:i32[])  [unwired: 2 in, 2 out]
            n266 = Insert Into Array(array=w408, index=w409, new element=1 ("new element/subarray")) -> (w406:i32[])
            n267 = property on="Selected\nCMF" class="Arr (strict)"() -> ("Value"=w405:dbl[][])  [unwired: 2 in, 2 out]
            n268 = call "CalculateXYZ.vi"("CMF"=w405, "Reflectance"=w406, "Illuminant"=w407) -> ()  [unwired: 1 out]
          }
        }
      }
    }
  }
